vi "Queued Pedestrian Lights Second Loop with FGV and use of Timeout.vi"() -> ()   [LabVIEW 2012]
doc: "Traffic Light VI with the use of Queues and LoadTrafficLightsQueue to Enqueue the Walk Element at the front of the initial State.\nNamed Second Loop as it uses second Loop to use an Event Structure with a Functional Global Boolean Variable to change the Waiting Indicator.\nTimeout Case has not been implemented at present."
uses:
  Controls/Traffic Light Display.ctl
  Controls/Pedestrian Light Display.ctl
  Controls/Traffic Light States (with Walk and Exit State).ctl
panel:
  out "Waiting":bool
  in  "Stop Button":bool
  out "Pedestrian Light Display":T1
  in  "Walk":bool
  out "Traffic Light Display":T2
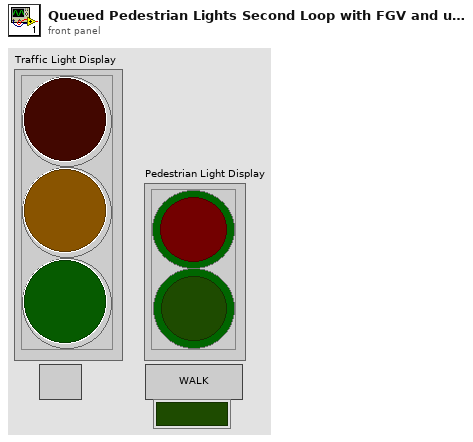
[diagram p1: front panel]
types:
  T1 = typedef "Pedestrian Light Display.ctl" = cluster{"Red":bool, "Green":bool}
  T2 = typedef "Traffic Light Display.ctl" = cluster{"RED":bool, "AMBER":bool, "GREEN":bool}
  T3 = typedef "Traffic Light States (with Walk and Exit State).ctl" = enum16{"Red", "RedAmber", "Green", "Amber", "Walk", "Exit"}
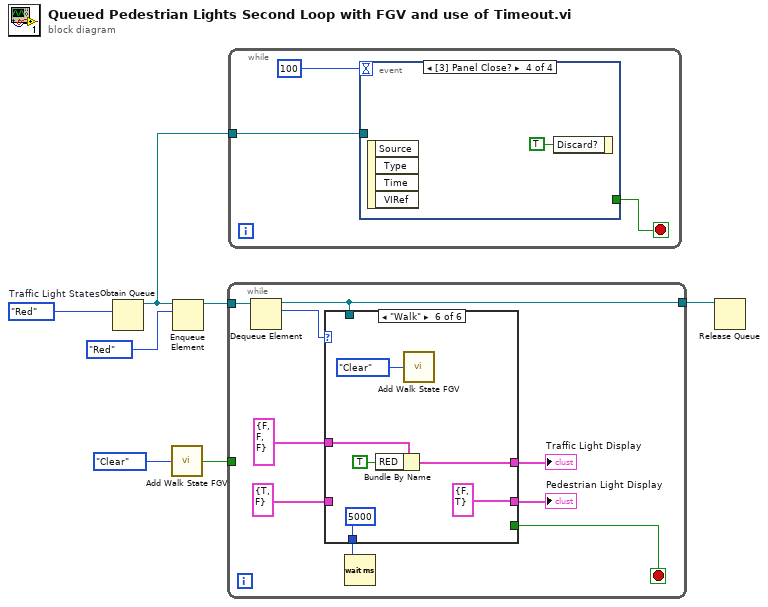
[diagram p0: block diagram]
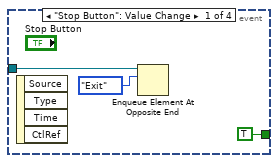
[diagram p2: hidden frame]
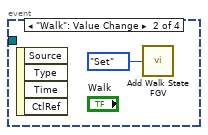
[diagram p3: hidden frame]
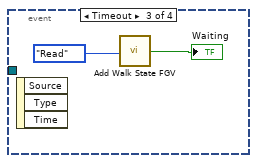
[diagram p4: hidden frame]
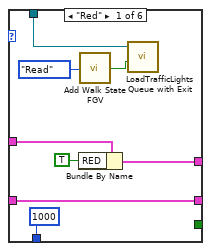
[diagram p5: hidden frame]
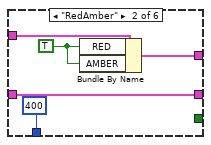
[diagram p6: hidden frame]
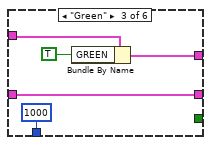
[diagram p7: hidden frame]
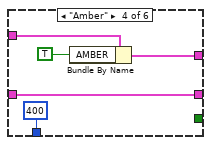
[diagram p8: hidden frame]
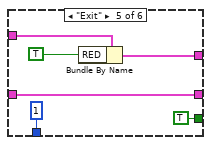
[diagram p9: hidden frame]
diagram:
  w4 = Traffic_Light_States_(with_Walk_and_Exit_State)."Red"  # Traffic Light States
  n1 = Obtain Queue(element data type=w4) -> (queue out=w6:refnum<queue>)  [unwired: 4 in, 2 out]
  n2 = call "Add Walk State FGV.vi"("FGV Function"=enum16{"Clear", "Set", "Read"}."Clear") -> ("Boolean Indicator"=w1:bool)
  n3 = Enqueue Element(queue=w6, element=Traffic_Light_States_(with_Walk_and_Exit_State)."Red" ("Traffic Light States")) -> (queue out=w7:refnum<queue>)  [unwired: 2 in, 2 out]
  n4 = while {
    tunnel: w7 -> [w11]
    tunnel: [w9] -> w5
    tunnel: w1 -> [_]
    stop <- w8 stop-if-true
    n5 = Dequeue Element(queue=w11) -> (queue out=w9:refnum<queue>, element=w10:T3)  [unwired: 2 in, 2 out]
    n6 = case shown="\"Walk\"" w10 {
      tunnel: T2 {"RED"=FALSE, "AMBER"=FALSE, "GREEN"=FALSE} ("Traffic Light Display") -> [w24 w29 w34 w39 w45 w50]
      tunnel: [w22 w28 w32 w37 w43 w48] -> w15
      tunnel: [1000 400 1000 400 1 5000] -> w14
      tunnel: T1 {"Red"=TRUE, "Green"=FALSE} ("Pedestrian Light Display") -> [w20 w26 w30 w35 w41 _]
      tunnel: [w20 w26 w30 w35 w41 T1 {"Red"=FALSE, "Green"=TRUE} ("Pedestrian Light Display")] -> w12
      tunnel: w9 -> [w17 _ _ _ _ _]
      tunnel: [_ _ _ _ TRUE _] -> w8
      frame "Red" {
        n7 = Bundle By Name(cluster=w24, "RED"=TRUE) -> (w22:T2)
        n8 = call "Add Walk State FGV.vi"("FGV Function"=enum16{"Clear", "Set", "Read"}."Read") -> ("Boolean Indicator"=w18:bool)
        n9 = call "LoadTrafficLightsQueue with Exit.vi"("Queue Ref in"=w17, "Walk"=w18) -> ()  [unwired: 9 in]
      }
      frame "RedAmber" {
        w25 = TRUE ("RED")
        n10 = Bundle By Name(cluster=w29, "RED"=w25, "AMBER"=w25) -> (w28:T2)
      }
      frame "Green" {
        n11 = Bundle By Name(cluster=w34, "GREEN"=TRUE ("RED")) -> (w32:T2)
      }
      frame "Amber" {
        n12 = Bundle By Name(cluster=w39, "AMBER"=TRUE ("RED")) -> (w37:T2)
      }
      frame "Exit" {
        n13 = Bundle By Name(cluster=w45, "RED"=TRUE) -> (w43:T2)
      }
      frame "Walk" {
        n14 = Bundle By Name(cluster=w50, "RED"=TRUE) -> (w48:T2)
        n15 = call "Add Walk State FGV.vi"("FGV Function"=enum16{"Clear", "Set", "Read"}."Clear") -> ()  [unwired: 1 out]
      }
    }
    "Traffic Light Display" <- w15
    "Pedestrian Light Display" <- w12
    n16 = Wait (ms)(milliseconds to wait=w14) -> ()  [unwired: 1 out]
  }
  n17 = while {
    tunnel: w6 -> [w53]
    stop <- w54 stop-if-true
    n18 = event shown="[3] Panel Close?" {
      selector: _ -> [_ _ _ _]
      dyn-events: _ -> [_ _ _ _]
      timeout: 100 -> [_ _ _ _]
      tunnel: [TRUE _ _ _] -> w54
      tunnel: w53 -> [w56 _ _ _]
      event "Stop Button": Value Change {
        n19 = event-data() -> ()  [unwired: 1 in, 4 out]
        n20 = Enqueue Element At Opposite End(queue=w56, element=Traffic_Light_States_(with_Walk_and_Exit_State)."Exit" ("Traffic Light States")) -> ()  [unwired: 2 in, 3 out]
      }
      event "Walk": Value Change {
        n21 = event-data() -> ()  [unwired: 1 in, 4 out]
        n22 = call "Add Walk State FGV.vi"("FGV Function"=enum16{"Clear", "Set", "Read"}."Set") -> ()  [unwired: 1 out]
      }
      event Timeout {
        n23 = event-data() -> ()  [unwired: 1 in, 3 out]
        n24 = call "Add Walk State FGV.vi"("FGV Function"=enum16{"Clear", "Set", "Read"}."Read") -> ("Boolean Indicator"=→"Waiting":bool)
      }
      event Panel Close? {
        n25 = event-data() -> ()  [unwired: 1 in, 4 out]
        n26 = event-data("Discard?"=TRUE) -> ()  [unwired: 1 in, 1 out]
      }
    }
  }
  n27 = Release Queue(queue=w5) -> ()  [unwired: 2 in, 3 out]
